vi "Status Notifiers.vi"() -> ()   [LabVIEW 2021]
uses:
  Globals and TypeDefs/Type Definitions.llb/McPherson Status.ctt
  Globals and TypeDefs/Type Definitions.llb/3 way Status.ctl
panel:
  in  "Spectrometer Pos":T2
  in  "notification":T3
  in  "PDA Exposure":u8(ring) items=["N.A.", "OK", "Busy", "Done"]
  out "Quit":bool
  in  "Status":string
  in  "Exp Index":u32
  in  "Saving":u8(ring) items=["N.A.", "OK", "Busy", "Done"]
  in  "Plotting":u8(ring) items=["N.A.", "OK", "Busy", "Done"]
  in  "Buffer":u8(ring) items=["N.A.", "OK", "Busy", "Done"]
  in  "CCD Exposure":u8(ring) items=["N.A.", "OK", "Busy", "Done"]
  in  "Spectrometer":u8(ring) items=["N.A.", "OK", "Busy", "Done"]
  in  "Temperature":u8(ring) items=["N.A.", "OK", "Busy", "Done"]
  in  "Field":u8(ring) items=["N.A.", "OK", "Busy", "Done"]
  in  "Time Between Iterations (ms)":u32=10
  in  "Stop":bool
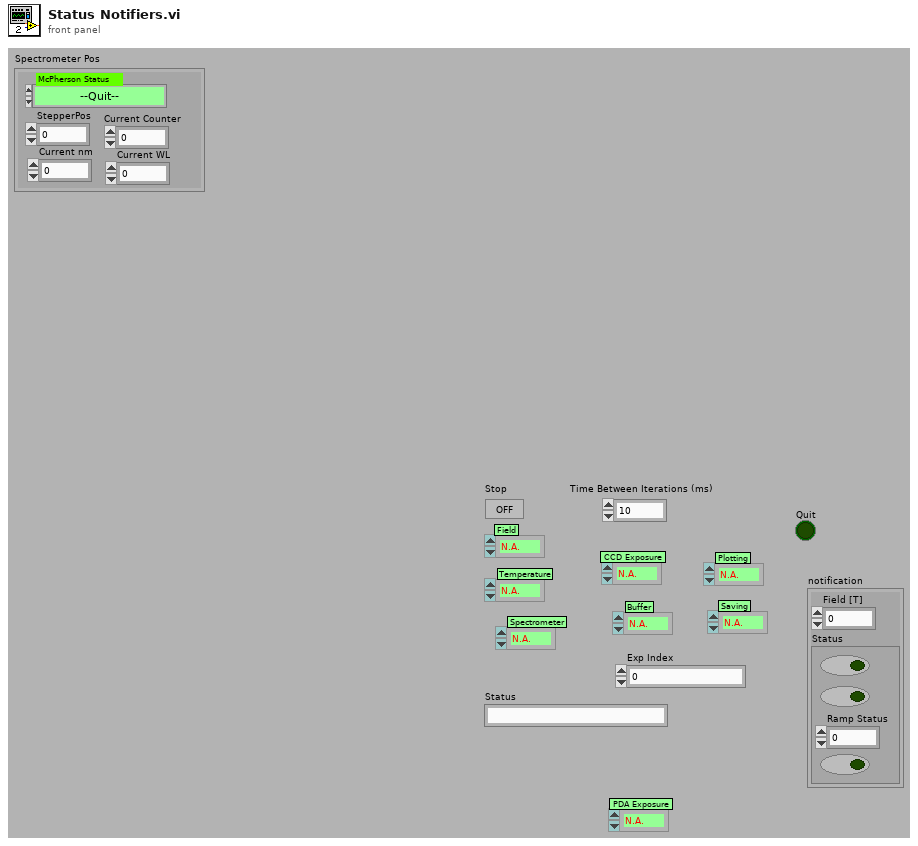
[diagram p1: front panel]
types:
  T1 = typedef "McPherson Status.ctt" = enum8{"--Quit--", "Error", "Initialization", "Standby", "Start Slew", "-Slew", "+Slew", "Slew Done", "Start Scan", "-Slew to Start", "+Slew to Start", "Scanning", "Scan Done", "Scan Pause", "Slew Pause", "Cancel", "Update Z0", "Sleep"}
  T2 = cluster{"StepperPos":i32, "Current nm":dbl, "Current Counter":dbl, "Current WL":dbl, "McPherson Status":T1}
  T3 = cluster{"Field [T]":dbl, "Status":cluster{bool, bool, "Ramp Status":u16, bool}}
  T4 = typedef "3 way Status.ctl" = u8
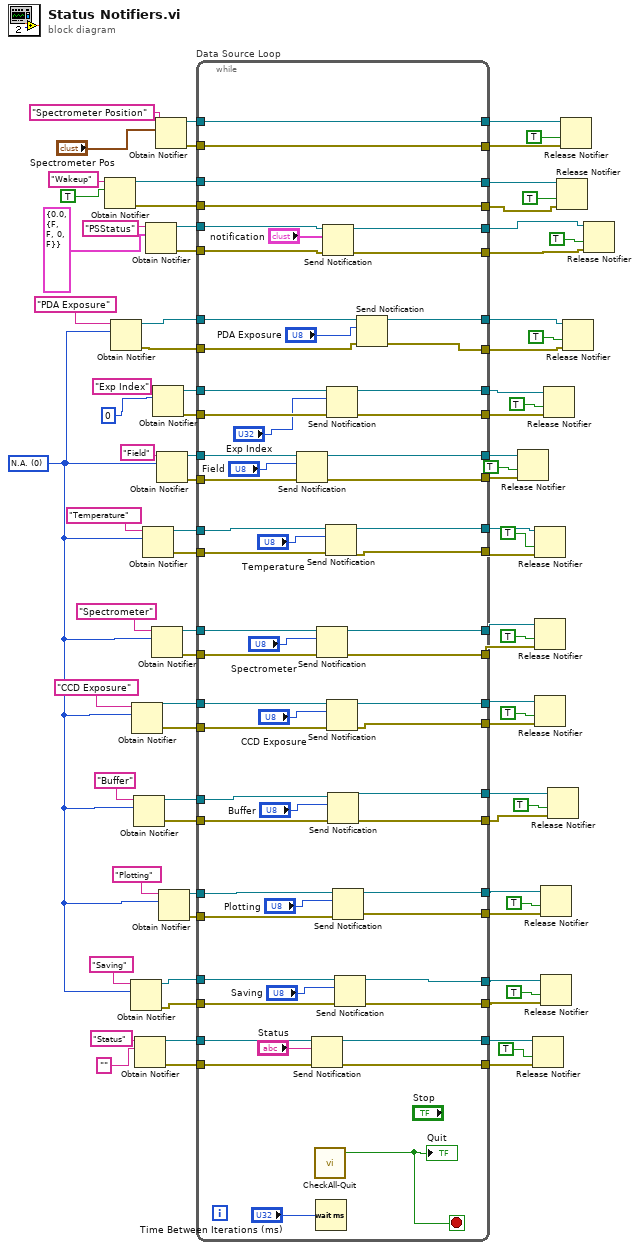
[diagram p0: block diagram]
diagram:
  w26 = T4 0 items=["N.A.", "OK", "Busy", "Done"] ("Saving")
  n1 = Obtain Notifier(name (unnamed)="Wakeup", notification data type=TRUE) -> (notifier out=w5:refnum<notifier>, error out=w4:errorcluster)  [unwired: 2 in, 1 out]
  n2 = Obtain Notifier(name (unnamed)="PDA Exposure", notification data type=w26) -> (notifier out=w25:refnum<notifier>, error out=w24:errorcluster)  [unwired: 2 in, 1 out]
  n3 = Obtain Notifier(name (unnamed)="Saving", notification data type=w26) -> (notifier out=w56:refnum<notifier>, error out=w55:errorcluster)  [unwired: 2 in, 1 out]
  n4 = Obtain Notifier(name (unnamed)="CCD Exposure", notification data type=w26) -> (notifier out=w61:refnum<notifier>, error out=w62:errorcluster)  [unwired: 2 in, 1 out]
  n5 = Obtain Notifier(name (unnamed)="Buffer", notification data type=w26) -> (notifier out=w60:refnum<notifier>, error out=w59:errorcluster)  [unwired: 2 in, 1 out]
  n6 = Obtain Notifier(name (unnamed)="Status", notification data type="" ("Status")) -> (notifier out=w32:refnum<notifier>, error out=w31:errorcluster)  [unwired: 2 in, 1 out]
  n7 = Obtain Notifier(name (unnamed)="Temperature", notification data type=w26) -> (notifier out=w66:refnum<notifier>, error out=w65:errorcluster)  [unwired: 2 in, 1 out]
  n8 = Obtain Notifier(name (unnamed)="PSStatus", notification data type=T3 {"Field [T]"=0.0, "Status"={FALSE, FALSE, "Ramp Status"=0, FALSE}} ("output cluster")) -> (notifier out=w18:refnum<notifier>, error out=w17:errorcluster)  [unwired: 2 in, 1 out]
  n9 = Obtain Notifier(name (unnamed)="Spectrometer", notification data type=w26) -> (notifier out=w64:refnum<notifier>, error out=w63:errorcluster)  [unwired: 2 in, 1 out]
  n10 = Obtain Notifier(name (unnamed)="Exp Index", notification data type=u32 0 ("Exp Index")) -> (notifier out=w40:refnum<notifier>, error out=w39:errorcluster)  [unwired: 2 in, 1 out]
  n11 = Obtain Notifier(name (unnamed)="Spectrometer Position", notification data type="Spectrometer Pos") -> (notifier out=w10:refnum<notifier>, error out=w9:errorcluster)  [unwired: 2 in, 1 out]
  n12 = Obtain Notifier(name (unnamed)="Field", notification data type=w26) -> (notifier out=w83:refnum<notifier>, error out=w82:errorcluster)  [unwired: 2 in, 1 out]
  n13 = Obtain Notifier(name (unnamed)="Plotting", notification data type=w26) -> (notifier out=w58:refnum<notifier>, error out=w57:errorcluster)  [unwired: 2 in, 1 out]
  n14 = while "Data Source Loop" {
    tunnel: w83 -> [w145]
    tunnel: w82 -> [w144]
    tunnel: [w143] -> w81
    tunnel: [w142] -> w80
    tunnel: w66 -> [w133]
    tunnel: w65 -> [w132]
    tunnel: w64 -> [w131]
    tunnel: w63 -> [w130]
    tunnel: w62 -> [w129]
    tunnel: w61 -> [w128]
    tunnel: w60 -> [w127]
    tunnel: w59 -> [w126]
    tunnel: w58 -> [w125]
    tunnel: w57 -> [w124]
    tunnel: w56 -> [w123]
    tunnel: w55 -> [w122]
    tunnel: [w121] -> w54
    tunnel: [w120] -> w53
    tunnel: [w119] -> w52
    tunnel: [w118] -> w51
    tunnel: [w117] -> w50
    tunnel: [w116] -> w49
    tunnel: [w115] -> w48
    tunnel: [w114] -> w47
    tunnel: [w113] -> w46
    tunnel: [w112] -> w45
    tunnel: [w111] -> w44
    tunnel: [w110] -> w43
    tunnel: w40 -> [w109]
    tunnel: w39 -> [w108]
    tunnel: [w107] -> w38
    tunnel: [w106] -> w37
    tunnel: w32 -> [w104]
    tunnel: w31 -> [w103]
    tunnel: [w102] -> w30
    tunnel: [w101] -> w29
    tunnel: w25 -> [w99]
    tunnel: w24 -> [w98]
    tunnel: [w96] -> w23
    tunnel: [w95] -> w22
    tunnel: w18 -> [w94]
    tunnel: w17 -> [w93]
    tunnel: [w92] -> w16
    tunnel: [w91] -> w15
    tunnel: [w89] -> w11
    tunnel: w10 -> [w89]
    tunnel: [w88] -> w8
    tunnel: w9 -> [w88]
    tunnel: [w87] -> w2
    tunnel: w5 -> [w87]
    tunnel: w4 -> [w86]
    tunnel: [w86] -> w1
    stop <- w85 stop-if-true
    n15 = Send Notification(notification="Field", notifier=w145, error in (no error)=w144) -> (notifier out=w143:refnum<notifier>, error out=w142:errorcluster)
    n16 = Send Notification(notification="Status", notifier=w104, error in (no error)=w103) -> (notifier out=w101:refnum<notifier>, error out=w102:errorcluster)
    n17 = call "CheckAll-Quit.vi"() -> ("All-Quit"=w85:bool)  [unwired: 3 in]
    "Quit" <- w85
    n18 = Wait (ms)(milliseconds to wait="Time Between Iterations (ms)") -> ()  [unwired: 1 out]
    n19 = Send Notification(notification="Spectrometer", notifier=w131, error in (no error)=w130) -> (notifier out=w119:refnum<notifier>, error out=w118:errorcluster)
    n20 = Send Notification(notification="notification", notifier=w94, error in (no error)=w93) -> (notifier out=w92:refnum<notifier>, error out=w91:errorcluster)
    n21 = Send Notification(notification="Temperature", notifier=w133, error in (no error)=w132) -> (notifier out=w120:refnum<notifier>, error out=w121:errorcluster)
    n22 = Send Notification(notification="Exp Index", notifier=w109, error in (no error)=w108) -> (notifier out=w106:refnum<notifier>, error out=w107:errorcluster)
    n23 = Send Notification(notification="CCD Exposure", notifier=w128, error in (no error)=w129) -> (notifier out=w117:refnum<notifier>, error out=w116:errorcluster)
    n24 = Send Notification(notification="Buffer", notifier=w127, error in (no error)=w126) -> (notifier out=w115:refnum<notifier>, error out=w114:errorcluster)
    n25 = Send Notification(notification="Plotting", notifier=w125, error in (no error)=w124) -> (notifier out=w113:refnum<notifier>, error out=w112:errorcluster)
    n26 = Send Notification(notification="Saving", notifier=w123, error in (no error)=w122) -> (notifier out=w111:refnum<notifier>, error out=w110:errorcluster)
    n27 = Send Notification(notification="PDA Exposure", notifier=w99, error in (no error)=w98) -> (notifier out=w96:refnum<notifier>, error out=w95:errorcluster)
  }
  n28 = Release Notifier(notifier=w81, force destroy? (F)=TRUE, error in (no error)=w80) -> ()  [unwired: 3 out]
  n29 = Release Notifier(notifier=w29, force destroy? (F)=TRUE, error in (no error)=w30) -> ()  [unwired: 3 out]
  n30 = Release Notifier(notifier=w53, force destroy? (F)=TRUE, error in (no error)=w54) -> ()  [unwired: 3 out]
  n31 = Release Notifier(notifier=w52, force destroy? (F)=TRUE, error in (no error)=w51) -> ()  [unwired: 3 out]
  n32 = Release Notifier(notifier=w50, force destroy? (F)=TRUE, error in (no error)=w49) -> ()  [unwired: 3 out]
  n33 = Release Notifier(notifier=w46, force destroy? (F)=TRUE, error in (no error)=w45) -> ()  [unwired: 3 out]
  n34 = Release Notifier(notifier=w44, force destroy? (F)=TRUE, error in (no error)=w43) -> ()  [unwired: 3 out]
  n35 = Release Notifier(notifier=w37, force destroy? (F)=TRUE, error in (no error)=w38) -> ()  [unwired: 3 out]
  n36 = Release Notifier(notifier=w48, force destroy? (F)=TRUE, error in (no error)=w47) -> ()  [unwired: 3 out]
  n37 = Release Notifier(notifier=w2, force destroy? (F)=TRUE, error in (no error)=w1) -> ()  [unwired: 3 out]
  n38 = Release Notifier(notifier=w11, force destroy? (F)=TRUE, error in (no error)=w8) -> ()  [unwired: 3 out]
  n39 = Release Notifier(notifier=w23, force destroy? (F)=TRUE, error in (no error)=w22) -> ()  [unwired: 3 out]
  n40 = Release Notifier(notifier=w16, force destroy? (F)=TRUE, error in (no error)=w15) -> ()  [unwired: 3 out]
